vi "toFile.vi"(5 "Temps t":i64, 6 "refnum":refnum<file>, 7 "entrée d'erreur":errorcluster, 8 "entree V":dbl, 9 "entree phi":dbl, 10 "sortie arr":dbl, 11 "sortie avant":dbl) -> (0 "refnum en sortie":refnum<file>, 3 "sortie d'erreur":errorcluster)   [LabVIEW 2019]
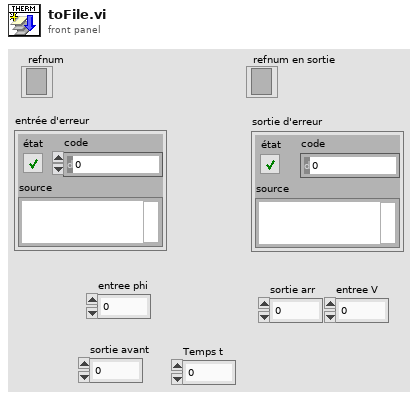
[diagram p1: front panel]
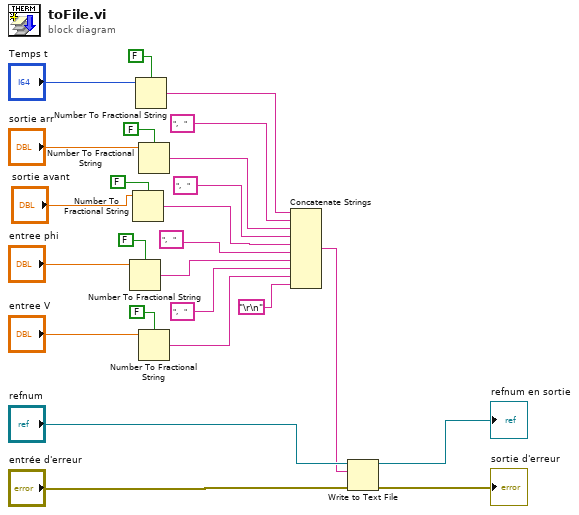
[diagram p0: block diagram]
diagram:
  n1 = Number To Fractional String(use system decimal point (T)=FALSE ("utiliser le séparateur décimal du système (V)"), number="entree phi") -> (F-format string=w10:string)  [unwired: 2 in]
  n2 = Number To Fractional String(use system decimal point (T)=FALSE ("utiliser le séparateur décimal du système (V)"), number="sortie avant") -> (F-format string=w3:string)  [unwired: 2 in]
  n3 = Number To Fractional String(use system decimal point (T)=FALSE ("utiliser le séparateur décimal du système (V)"), number="Temps t") -> (F-format string=w7:string)  [unwired: 2 in]
  n4 = Number To Fractional String(use system decimal point (T)=FALSE ("utiliser le séparateur décimal du système (V)"), number="sortie arr") -> (F-format string=w5:string)  [unwired: 2 in]
  n5 = Number To Fractional String(use system decimal point (T)=FALSE ("utiliser le séparateur décimal du système (V)"), number="entree V") -> (F-format string=w19:string)  [unwired: 2 in]
  n6 = Concatenate Strings(w7, ",   " ("chaîne"), w5, ",   " ("chaîne"), w3, ",   " ("chaîne"), w10, ",   " ("chaîne"), w19, "\r\n") -> (w20:string)
  n7 = Write to Text File(file (use dialog)="refnum", text=w20, error in="entrée d'erreur") -> (refnum out=→"refnum en sortie":refnum<file>, error out=→"sortie d'erreur":errorcluster)  [unwired: 1 in, 1 out]
